vi "playLongestSequence.vi"(8 "error in (no error)":errorcluster, 11 "Simon_Engine in":refnum<class "Simon_Engine.lvclass">) -> (0 "error out":errorcluster, 3 "Simon_Engine out":refnum<class "Simon_Engine.lvclass">)   [LabVIEW 2019, in "Simon_Engine.lvclass"]
uses:
  Simon_Engine.lvclass
  LED/LED Class/LED.lvclass
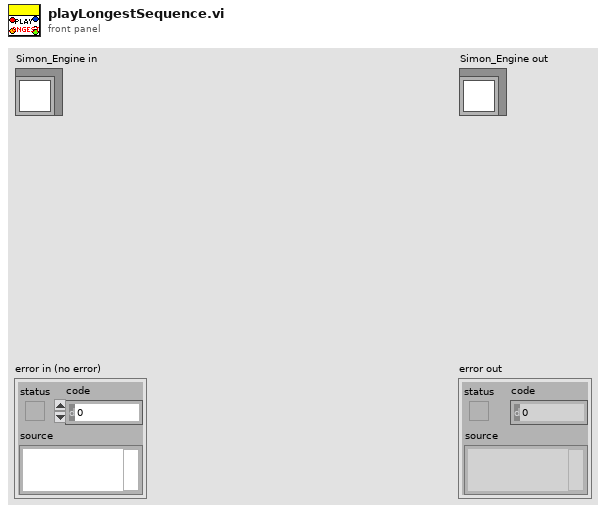
[diagram p1: front panel]
types:
  T1 = enum8{"Enabled", "Disabled", "Disabled and Grayed Out"}
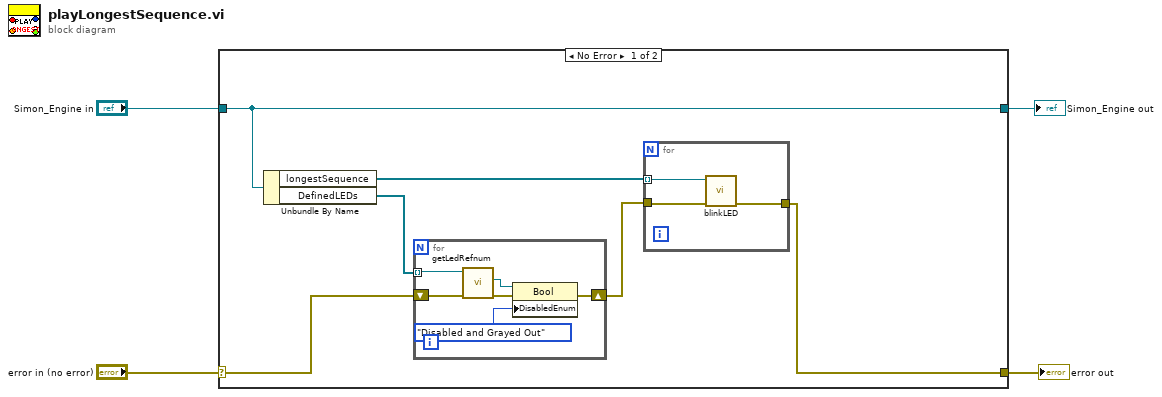
[diagram p0: block diagram]
diagram:
  n1 = case shown="No Error" "error in (no error)" {
    selector: "error in (no error)" -> [w6 w21]
    tunnel: [w9 w21] -> w3
    tunnel: [w5 w20] -> w1
    tunnel: "Simon_Engine in" -> [w5 w20]
    frame No Error {
      n2 = Unbundle By Name(w5) -> ("longestSequence"=w10:refnum<class "LED.lvclass">[], "DefinedLEDs"=w7:refnum<class "LED.lvclass">[])
      n3 = for {
        shift-right: [w15] -> w8
        shift-left: w6 -> [w16]
        tunnel: w7 -> [w13] mode=indexing
        n4 = call "getLedRefnum.vi"("error in (no error)"=w16, "LED in"=w13) -> ("error out"=w14:errorcluster, "LED Refnum"=w12:refnum<vi>)  [unwired: 7 in, 1 out]
        n5 = property class="Bool"(reference=w12, error in=w14, "DisabledEnum"=T1."Disabled and Grayed Out" ("Disabled")) -> (error out=w15:errorcluster)  [unwired: 1 out]
      }
      n6 = for {
        tunnel: w10 -> [w19] mode=indexing
        tunnel: w8 -> [w18]
        tunnel: [w17] -> w9
        n7 = call "blinkLED.vi"("error in (no error)"=w18, "LED in"=w19) -> ("error out"=w17:errorcluster)  [unwired: 8 in, 1 out]
      }
    }
    frame Error {
    }
  }
  "error out" <- w3
  "Simon_Engine out" <- w1
